vi "Aliases Definition Window.vi"() -> ()   [LabVIEW 2021, in "Formula.lvlib"]
uses:
  Formula.lvlib
  Alias Definition Q Element.ctl
  Alias Definition Q Action.ctl
  Formula Alias Definition.ctl
panel:
  in  "Send New Definitions to Notebook":bool=TRUE
  in  "Alias Description":string
  in  "Load Aliases":bool
  in  "Save Aliases":bool
  out "Invalid Alias":bool
  out "Invalid Formula":bool
  in  "Alias Name":string
  in  "Remove Alias":bool
  in  "Add/Modify Alias":bool
  in  "Alias Definition":string
  in  "Aliases List":i32[](listbox)
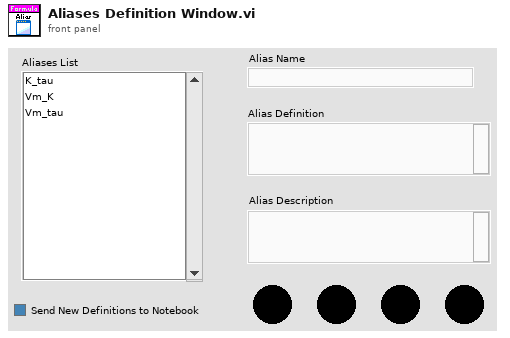
[diagram p1: front panel]
types:
  T1 = typedef "Formula.lvlib/Alias Definition Q Element.ctl" = cluster{"Action":T2, "Data":variant}
  T2 = typedef "Formula.lvlib/Alias Definition Q Action.ctl" = enum16{"Idle", "Check Alias Name", "Get Alias Definition", "Add Alias", "Remove Alias", "Save Alias Definitions", "Load Alias Definitions", "Sort Aliases", "Send Selected Aliases to Notebook", "Quit"}
  T3 = typedef "Formula.lvlib/Formula Alias Definition.ctl" = cluster{"Alias Formula":string, "Alias Name":string, "Alias Description":string}
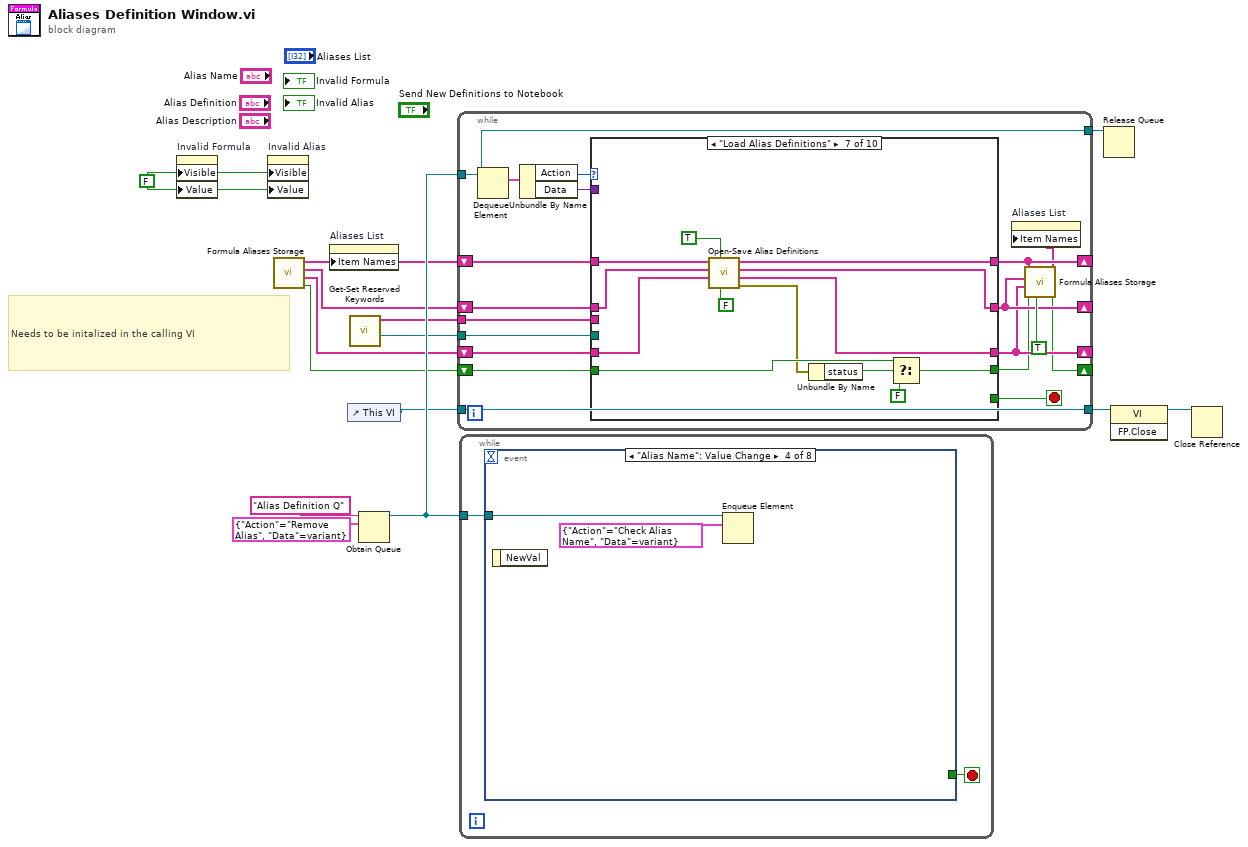
[diagram p0: block diagram]
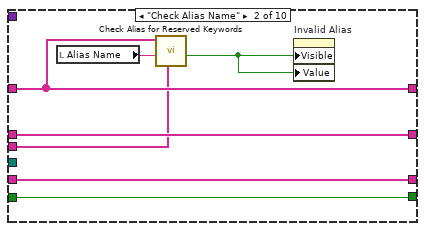
[diagram p3: hidden frame]
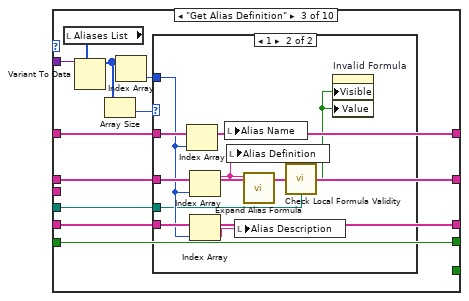
[diagram p4: hidden frame]
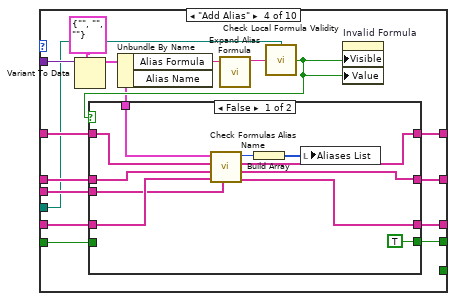
[diagram p6: hidden frame]
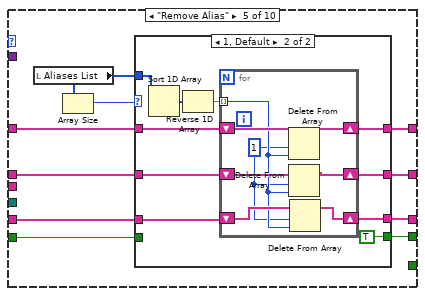
[diagram p8: hidden frame]
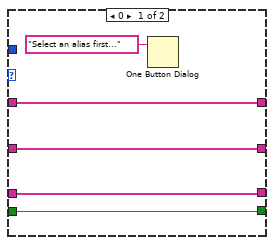
[diagram p9: hidden frame]
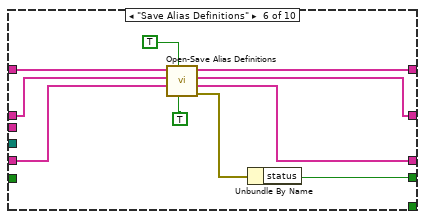
[diagram p10: hidden frame]
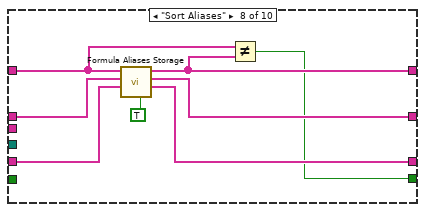
[diagram p11: hidden frame]
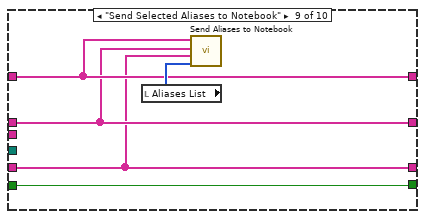
[diagram p12: hidden frame]
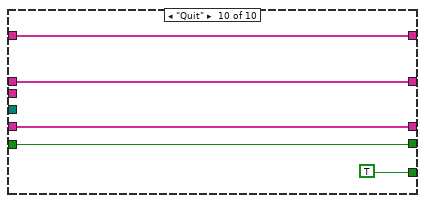
[diagram p13: hidden frame]
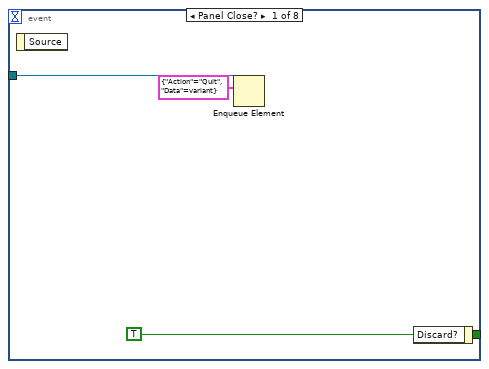
[diagram p14: hidden frame]
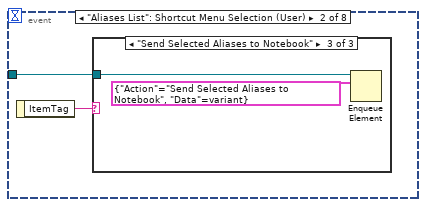
[diagram p15: hidden frame]
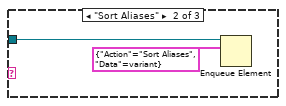
[diagram p17: hidden frame]
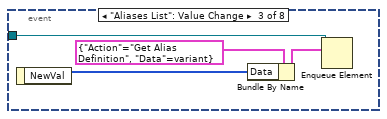
[diagram p18: hidden frame]
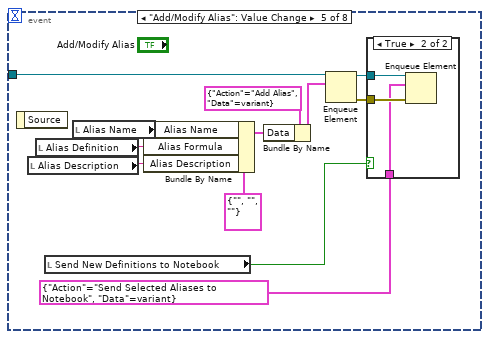
[diagram p19: hidden frame]
diagram:
  w8 = FALSE ("Valid Formula?")
  # "Needs to be initalized in the calling VI"
  n1 = property on="Invalid Formula" class="Bool (strict)"("Visible"=w8, "Value"=w8) -> ()  [unwired: 2 in, 2 out]
  n2 = property on="Invalid Alias" class="Bool (strict)"("Visible"=w8, "Value"=w8) -> ()  [unwired: 2 in, 2 out]
  n3 = call "Formula Aliases Storage.vi"() -> ("Alias list modified since last saved"=w5:bool, "Descriptions Array"=w6:string[], "Definitions Array"=w7:string[], "Aliases Array"=w10:string[])  [unwired: 8 in]
  n4 = property on="Aliases List" class="LstBox (strict)"("Item Names"=w10) -> ()  [unwired: 2 in, 2 out]
  n5 = control-ref of="This VI"() -> (w3:refnum<vi>)
  n6 = call "Get-Set Reserved Keywords.vi"() -> ("Formula Interpreter Path"=w1:path, "Reserved Keywords"=w2:string[])  [unwired: 9 in, 1 out]
  n7 = Obtain Queue(name (unnamed)="Alias Definition Q", element data type=T1 {"Action"=enum."Remove Alias", "Data"=variant}) -> (queue out=w12:refnum<queue>)  [unwired: 3 in, 2 out]
  n8 = while {
    tunnel: w12 -> [w21]
    tunnel: [w21] -> w11
    shift-right: [w27] -> _
    shift-left: w10 -> [w29]
    shift-right: [w23] -> _
    shift-left: w7 -> [w28]
    shift-right: [w22] -> _
    shift-left: w6 -> [w24]
    shift-right: [w19] -> _
    shift-left: w5 -> [w18]
    tunnel: [w17] -> w4
    tunnel: w3 -> [w17]
    tunnel: w2 -> [w16]
    tunnel: w1 -> [w15]
    stop <- w31 stop-if-true
    n9 = Dequeue Element(queue=w21) -> (element=w33:T1)  [unwired: 2 in, 3 out]
    n10 = Unbundle By Name(w33) -> ("Action"=w32:T2, "Data"=w30:variant)
    n11 = case shown="\"Load Alias Definitions\"" w32 {
      tunnel: [_ _ _ _ _ _ _ _ _ TRUE] -> w31
      tunnel: w30 -> [_ _ w54 w80 _ _ _ _ _ _]
      tunnel: w29 -> [w37 w42 w52 w77 w105 w138 w151 w154 w163 w169]
      tunnel: w28 -> [w36 w43 w53 w76 w104 w137 w150 w158 w162 w168]
      tunnel: [w37 w42 w52 w75 w103 w136 w149 w153 w163 w169] -> w27
      tunnel: [w36 w43 w53 w74 w102 w135 w148 w157 w162 w168] -> w23
      tunnel: w24 -> [w35 w41 w47 w70 w99 w133 w146 w156 w161 w167]
      tunnel: [w35 w41 w47 w69 w98 w132 w145 w155 w161 w167] -> w22
      tunnel: [w34 w40 w46 w68 w97 w131 w142 w152 w160 w165] -> w20
      tunnel: w18 -> [w34 w40 w46 w67 w96 _ w143 _ w160 w165]
      tunnel: w16 -> [_ w38 _ w66 _ _ _ _ _ _]
      tunnel: w15 -> [_ _ w45 w65 _ _ _ _ _ _]
      frame "Idle", Default {
      }
      frame "Check Alias Name" {
        n12 = local read "Alias Name"() -> (w39:string)
        n13 = call "Check Alias for Reserved Keywords.vi"("Reserved Keywords"=w38, "Alias Name"=w39, "Aliases Array in"=w42) -> ("Is Part of Reserved Keywords"=w44:bool)  [unwired: 5 in, 3 out]
        n14 = property on="Invalid Alias" class="Bool (strict)"("Visible"=w44, "Value"=w44) -> ()  [unwired: 2 in, 2 out]
      }
      frame "Get Alias Definition" {
        n15 = local read "Aliases List"() -> (w51:i32[])
        n16 = Variant To Data(type=w51, Variant=w54) -> (data=w49:i32[])  [unwired: 1 in, 1 out]
        n17 = Array Size(array=w49) -> (size(s)=w50:i32)
        n18 = Index Array(array=w49) -> (element=w48:i32)  [unwired: 1 in]
        n19 = case shown="1" w50 {
          tunnel: w53 -> [_ w64]
          tunnel: w52 -> [_ w63]
          tunnel: w48 -> [_ w57]
          tunnel: w47 -> [_ w58]
          tunnel: w45 -> [_ w55]
          frame 0, Default {
          }
          frame 1 {
            n20 = Index Array(array=w63, index=w57) -> (element=w62:string)
            n21 = Index Array(array=w64, index=w57) -> (element=w59:string)
            n22 = Index Array(array=w58, index=w57) -> (element=w56:string)
            n23 = local write "Alias Name"(w62) -> ()
            n24 = local write "Alias Definition"(w59) -> ()
            n25 = local write "Alias Description"(w56) -> ()
            n26 = call "Expand Alias Formula.vi"("Alias Definition in"=w59) -> ("Expanded Alias Definition out"=w61:string)  [unwired: 10 in]
            n27 = call "Check Local Formula Validity.vi"("Fornula"=w61, "Formula Interpreter's Path"=w55) -> ("Error?"=w60:bool)  [unwired: 13 in]
            n28 = property on="Invalid Formula" class="Bool (strict)"("Visible"=w60, "Value"=w60) -> ()  [unwired: 2 in, 2 out]
          }
        }
      }
      frame "Add Alias" {
        n29 = Variant To Data(type=T3 {"Alias Formula"="", "Alias Name"="", "Alias Description"=""} ("Alias Definition"), Variant=w80) -> (data=w71:T3)  [unwired: 1 in, 1 out]
        n30 = Unbundle By Name(w71) -> ("Alias Formula"=w73:string)  [unwired: 1 out]
        n31 = call "Expand Alias Formula.vi"("Alias Definition in"=w73) -> ("Expanded Alias Definition out"=w78:string)  [unwired: 10 in]
        n32 = call "Check Local Formula Validity.vi"("Fornula"=w78, "Formula Interpreter's Path"=w65) -> ("Error?"=w72:bool)  [unwired: 13 in]
        n33 = case shown="False" w72 {
          tunnel: w77 -> [w88 w95]
          tunnel: w76 -> [w87 w94]
          tunnel: [w85 w95] -> w75
          tunnel: [w84 w94] -> w74
          tunnel: w71 -> [w89 _]
          tunnel: w70 -> [w86 w93]
          tunnel: [w83 w93] -> w69
          tunnel: [TRUE ("Aliases modified since saved") w92] -> w68
          tunnel: w67 -> [_ w92]
          tunnel: w66 -> [w81 _]
          frame False {
            n34 = call "Check Formulas Alias Name.vi"("Reserved Keywords"=w81, "Descriptions Array in"=w86, "Definitions Array in"=w87, "Aliases Array in"=w88, "Alias Definition"=w89) -> ("Descriptions Array out"=w83:string[], "Definitions Array out"=w84:string[], "Aliases Array out"=w85:string[], "Selected Alias"=w91:i32)  [unwired: 3 in]
            n35 = Build Array(w91) -> (w90:i32[])
            n36 = local write "Aliases List"(w90) -> ()
          }
          frame True {
            # "Not a valid formula"
          }
        }
        n37 = property on="Invalid Formula" class="Bool (strict)"("Visible"=w72, "Value"=w72) -> ()  [unwired: 2 in, 2 out]
      }
      frame "Remove Alias" {
        n38 = local read "Aliases List"() -> (w100:i32[])
        n39 = Array Size(array=w100) -> (size(s)=w101:i32)
        n40 = case shown="1, Default" w101 {
          tunnel: w105 -> [w109 w120]
          tunnel: w104 -> [w108 w118]
          tunnel: [w109 w119] -> w103
          tunnel: [w108 w117] -> w102
          tunnel: w100 -> [_ w116]
          tunnel: w99 -> [w107 w113]
          tunnel: [w107 w112] -> w98
          tunnel: [w106 TRUE ("Aliases modified since saved")] -> w97
          tunnel: w96 -> [w106 _]
          frame 0 {
            n41 = One Button Dialog(message="Select an alias first...") -> ()  [unwired: 1 in, 1 out]
          }
          frame 1, Default {
            n42 = Sort 1D Array(array=w116) -> (sorted array=w115:i32[])
            n43 = Reverse 1D Array(array=w115) -> (reversed array=w114:i32[])
            n44 = for {
              tunnel: w114 -> [w122] mode=indexing
              shift-right: [w127] -> w119
              shift-left: w120 -> [w128]
              shift-right: [w125] -> w117
              shift-left: w118 -> [w126]
              shift-right: [w123] -> w112
              shift-left: w113 -> [w124]
              w121 = 1 ("length")
              n45 = Delete From Array(array=w128, length=w121, index=w122) -> (array with subset deleted=w127:string[])  [unwired: 1 out]
              n46 = Delete From Array(array=w126, length=w121, index=w122) -> (array with subset deleted=w125:string[])  [unwired: 1 out]
              n47 = Delete From Array(array=w124, length=w121, index=w122) -> (array with subset deleted=w123:string[])  [unwired: 1 out]
            }
          }
        }
      }
      frame "Save Alias Definitions" {
        n48 = call "Open-Save Alias Definitions.vi"("Open (F)/ Save"=TRUE, "Dialog? (F)"=TRUE, "Descriptions Array in"=w133, "Definitions Array in"=w137, "Aliases Array in"=w138) -> ("Error Out"=w130:errorcluster, "Descriptions Array out"=w132:string[], "Definitions Array out"=w135:string[], "Aliases Array out"=w136:string[])  [unwired: 2 in, 1 out]
        n49 = Unbundle By Name(w130) -> ("status"=w131:bool)
      }
      frame "Load Alias Definitions" {
        n50 = call "Open-Save Alias Definitions.vi"("Open (F)/ Save"=FALSE, "Dialog? (F)"=TRUE, "Descriptions Array in"=w146, "Definitions Array in"=w150, "Aliases Array in"=w151) -> ("Error Out"=w140:errorcluster, "Descriptions Array out"=w145:string[], "Definitions Array out"=w148:string[], "Aliases Array out"=w149:string[])  [unwired: 2 in, 1 out]
        n51 = Unbundle By Name(w140) -> ("status"=w144:bool)
        n52 = Select(t=w143, s=w144, f=FALSE) -> (s? t:f=w142:bool)
      }
      frame "Sort Aliases" {
        n53 = call "Formula Aliases Storage.vi"("Sort"=TRUE, "Descriptions Array in"=w156, "Definitions Array in"=w158, "Aliases Array in"=w154) -> ("Descriptions Array"=w155:string[], "Definitions Array"=w157:string[], "Aliases Array"=w153:string[])  [unwired: 4 in, 1 out]
        n54 = Not Equal?(x=w154, y=w153) -> (x != y?=w152:bool)
      }
      frame "Send Selected Aliases to Notebook" {
        n55 = local read "Aliases List"() -> (w164:i32[])
        n56 = call "Send Aliases to Notebook.vi"("Satistics Aliases"=w164, "Descriptions Array"=w161, "Definitions Array"=w162, "Aliases Array"=w163) -> ()  [unwired: 8 in]
      }
      frame "Quit" {
      }
    }
    n57 = call "Formula Aliases Storage.vi"("Get (F)/Set"=TRUE, "Alias list modified since last saved"=w20, "Descriptions Array in"=w22, "Definitions Array in"=w23, "Aliases Array in"=w27) -> ("Alias list modified since last saved"=w19:bool, "Aliases Array"=w25:string[])  [unwired: 3 in, 2 out]
    n58 = property on="Aliases List" class="LstBox (strict)"("Item Names"=w25) -> ()  [unwired: 2 in, 2 out]
  }
  n59 = while {
    tunnel: w12 -> [w170]
    stop <- w171 stop-if-true
    n60 = event shown="[3] \"Alias Name\": Value Change" {
      selector: _ -> [_ _ _ _ _ _ _ _]
      dyn-events: _ -> [_ _ _ _ _ _ _ _]
      timeout: _ -> [_ _ _ _ _ _ _ _]
      tunnel: [w174 _ _ _ _ _ _ _] -> w171
      tunnel: w170 -> [w173 w175 w184 w186 w198 w203 w205 w207]
      event Panel Close? {
        w174 = TRUE ("Discard?")
        n61 = event-data() -> ()  [unwired: 1 in, 1 out]
        n62 = Enqueue Element(queue=w173, element=T1 {"Action"=enum."Quit", "Data"=variant}) -> ()  [unwired: 2 in, 3 out]
        n63 = event-data("Discard?"=w174) -> ()  [unwired: 1 in, 1 out]
      }
      event "Aliases List": Shortcut Menu Selection (User) {
        n64 = event-data() -> ("ItemTag"=w176:string)  [unwired: 1 in]
        n65 = case shown="\"Send Selected Aliases to Notebook\"" w176 {
          tunnel: w175 -> [_ w178 w180]
          frame "", Default {
          }
          frame "Sort Aliases" {
            n66 = Enqueue Element(queue=w178, element=T1 {"Action"=enum."Sort Aliases", "Data"=variant}) -> ()  [unwired: 2 in, 3 out]
          }
          frame "Send Selected Aliases to Notebook" {
            n67 = Enqueue Element(queue=w180, element=T1 {"Action"=enum."Send Selected Aliases to Notebook", "Data"=variant}) -> ()  [unwired: 2 in, 3 out]
          }
        }
      }
      event "Aliases List": Value Change {
        n68 = event-data() -> ("NewVal"=w181:i32[])  [unwired: 1 in]
        n69 = Bundle By Name(cluster=T1 {"Action"=enum."Get Alias Definition", "Data"=variant} ("element"), "Data"=w181) -> (w182:T1)
        n70 = Enqueue Element(queue=w184, element=w182) -> ()  [unwired: 2 in, 3 out]
      }
      event "Alias Name": Value Change {
        n71 = event-data() -> ()  [unwired: 1 in, 1 out]
        n72 = Enqueue Element(queue=w186, element=T1 {"Action"=enum."Check Alias Name", "Data"=variant}) -> ()  [unwired: 2 in, 3 out]
      }
      event "Add/Modify Alias": Value Change {
        n73 = event-data() -> ()  [unwired: 1 in, 1 out]
        n74 = local read "Alias Description"() -> (w191:string)
        n75 = local read "Alias Definition"() -> (w192:string)
        n76 = local read "Send New Definitions to Notebook"() -> (w190:bool)
        n77 = local read "Alias Name"() -> (w193:string)
        n78 = Bundle By Name(cluster=T3 {"Alias Formula"="", "Alias Name"="", "Alias Description"=""} ("Alias Definition"), "Alias Name"=w193, "Alias Formula"=w192, "Alias Description"=w191) -> (w194:T3)
        n79 = Bundle By Name(cluster=T1 {"Action"=enum."Add Alias", "Data"=variant} ("element"), "Data"=w194) -> (w196:T1)
        n80 = Enqueue Element(queue=w198, element=w196) -> (queue out=w189:refnum<queue>, error out=w188:errorcluster)  [unwired: 2 in, 1 out]
        n81 = case shown="True" w190 {
          tunnel: w189 -> [_ w201]
          tunnel: w188 -> [_ w200]
          tunnel: T1 {"Action"=enum."Send Selected Aliases to Notebook", "Data"=variant} ("element") -> [_ w199]
          frame False {
          }
          frame True {
            n82 = Enqueue Element(queue=w201, element=w199, error in (no error)=w200) -> ()  [unwired: 1 in, 3 out]
          }
        }
      }
      event "Remove Alias": Value Change {
        n83 = event-data() -> ()  [unwired: 1 in, 1 out]
        n84 = Enqueue Element(queue=w203, element=T1 {"Action"=enum."Remove Alias", "Data"=variant}) -> ()  [unwired: 2 in, 3 out]
      }
      event "Save Aliases": Value Change {
        n85 = event-data() -> ()  [unwired: 1 in, 1 out]
        n86 = Enqueue Element(queue=w205, element=T1 {"Action"=enum."Save Alias Definitions", "Data"=variant}) -> ()  [unwired: 2 in, 3 out]
      }
      event "Load Aliases": Value Change {
        n87 = event-data() -> ()  [unwired: 1 in, 1 out]
        n88 = Enqueue Element(queue=w207, element=T1 {"Action"=enum."Load Alias Definitions", "Data"=variant}) -> ()  [unwired: 2 in, 3 out]
      }
    }
  }
  n89 = Release Queue(queue=w11) -> ()  [unwired: 2 in, 3 out]
  n90 = invoke class="VI" method="FP.Close"(reference=w4) -> (reference out=w9:refnum<vi>)  [unwired: 2 in, 2 out]
  n91 = Close Reference(reference=w9) -> ()  [unwired: 1 in, 1 out]
